vi "Чтение волны.vi"() -> ()   [LabVIEW 2017]
panel:
  in  "stop":bool
  out "Waveform Chart":cluster{dbl, dbl}(graph)
  in  "file path (use dialog)":path
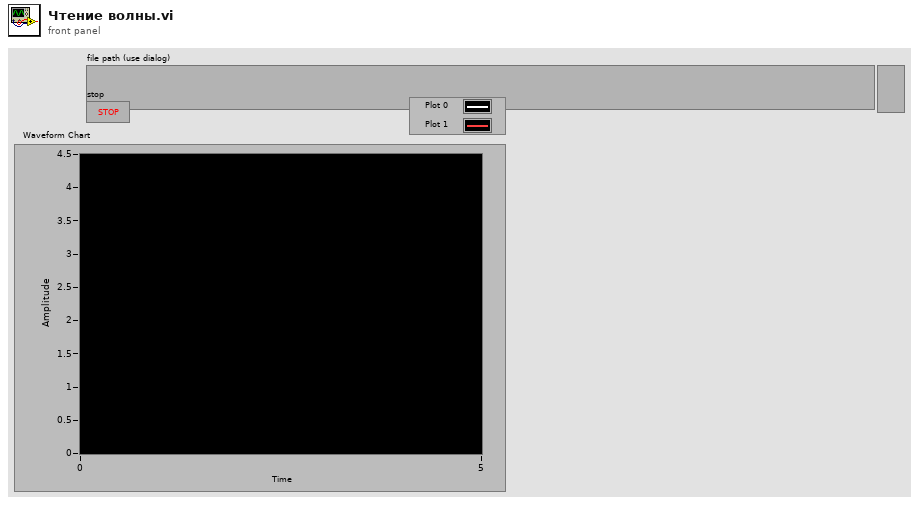
[diagram p1: front panel]
types:
  T1 = enum16{"open", "replace", "create", "open or create", "replace or create", "replace or create with confirmation"}
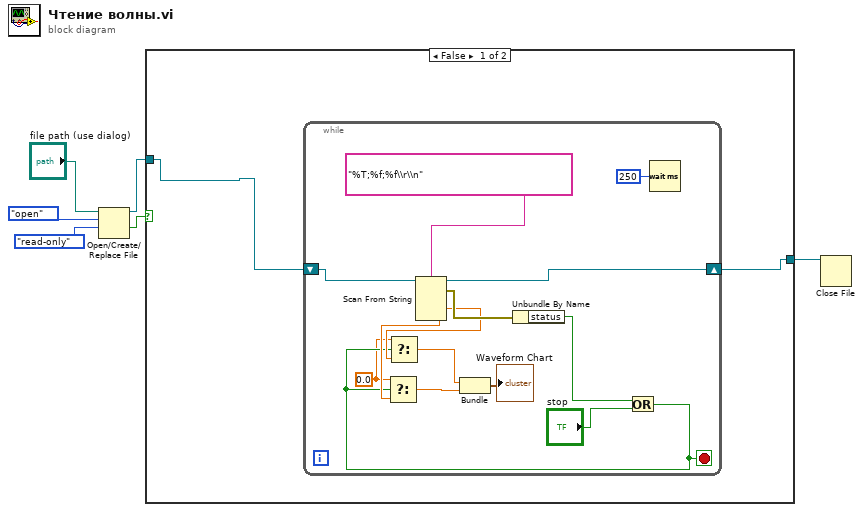
[diagram p0: block diagram]
diagram:
  n1 = Open/Create/Replace File(file path (use dialog)="file path (use dialog)", operation (0:open)=T1."open", access (0:read/write)=enum16{"read/write", "read-only", "write-only"}."read-only") -> (refnum out=w2:refnum<file>, cancelled=w3:bool)  [unwired: 3 in, 1 out]
  n2 = case shown="False" w3 {
    tunnel: w2 -> [w7 w23]
    tunnel: [w8 w23] -> w1
    frame False {
      n3 = while {
        shift-right: [w20] -> w8
        shift-left: w7 -> [w22]
        stop <- w11 stop-if-true
        w10 = 0.0 ("t")
        n4 = Scan From String("%T;%f;%f\\r\\n" ("format string"), w22) -> (w20:refnum<file>, w19:errorcluster, output 2=w13:dbl, output 3=w12:dbl)  [unwired: 5 in]
        n5 = Unbundle By Name(w19) -> ("status"=w17:bool)
        n6 = Or(x=w17, y="stop") -> (x .or. y?=w11:bool)
        n7 = Select(t=w10, s=w11, f=w12) -> (s? t:f=w15:dbl)
        n8 = Select(t=w10, s=w11, f=w13) -> (s? t:f=w14:dbl)
        n9 = Bundle("t"=w14, "t"=w15) -> (→"Waveform Chart":cluster{"t":dbl, "t":dbl})  [unwired: 1 in]
        n10 = Wait (ms)(milliseconds to wait=u32 250) -> ()  [unwired: 1 out]
      }
    }
    frame True {
    }
  }
  n11 = Close File(refnum=w1) -> ()  [unwired: 1 in, 2 out]
